vi "Level.vi"(0 "In":dbl, 1 "In 2":dbl) -> (6 "Boolean":bool)   [LabVIEW 2015]
panel:
  out "Boolean 2":bool
  in  "Thresh":dbl=6.0
  in  "DB_Count":dbl
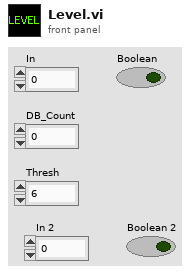
[diagram p1: front panel]
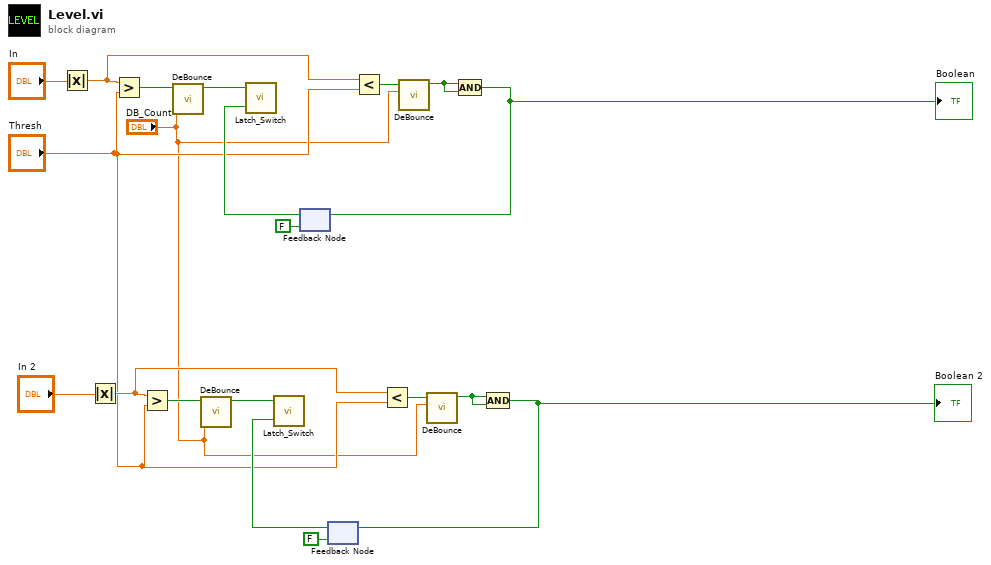
[diagram p0: block diagram]
diagram:
  n1 = Absolute Value(x="In") -> (abs(x)=w14:dbl)
  n2 = Absolute Value(x="In 2") -> (abs(x)=w9:dbl)
  n3 = Greater?(x=w14, y="Thresh") -> (0:w18:bool)
  n4 = Greater?(x=w9, y="Thresh") -> (0:w5:bool)
  n5 = call "DeBounce.vi"("DB_Count"="DB_Count", "Value"=w18) -> ("BD_Value"=w19:bool)  [unwired: 9 in]
  n6 = call "DeBounce.vi"("DB_Count"="DB_Count", "Value"=w5) -> ("BD_Value"=w4:bool)  [unwired: 9 in]
  n7 = feedback #1(FALSE) -> (w17:bool)
  n8 = call "Latch_Switch.vi"("Reset"=w17, "In"=w19) -> ()  [unwired: 1 out]
  n9 = feedback #2(FALSE) -> (w6:bool)
  n10 = call "Latch_Switch.vi"("Reset"=w6, "In"=w4) -> ()  [unwired: 1 out]
  n11 = Less?(x=w14, y="Thresh") -> (x < y?=w20:bool)
  n12 = Less?(x=w9, y="Thresh") -> (x < y?=w3:bool)
  n13 = call "DeBounce.vi"("DB_Count"="DB_Count", "Value"=w20) -> ("BD_Value"=w12:bool)  [unwired: 9 in]
  n14 = call "DeBounce.vi"("DB_Count"="DB_Count", "Value"=w3) -> ("BD_Value"=w11:bool)  [unwired: 9 in]
  n15 = Compound Arithmetic op=AND(w12, w12) -> (w16:bool)
  "Boolean" <- w16
  n16 = feedback-in #1(w16) -> ()
  n17 = Compound Arithmetic op=AND(w11, w11) -> (w7:bool)
  "Boolean 2" <- w7
  n18 = feedback-in #2(w7) -> ()
